vi "AdditiveChi2Sampler.vi"(8 "error in":errorcluster caption="entrée d'erreur", 11 "AdditiveChi2Sampler":T1={"sample_steps"=2, "sample_interval"=-1.0} {"sample_interval" min=-1.0}) -> (0 "error out":errorcluster caption="sortie d'erreur", 3 "AdditiveChi2Sampler.lvclass":refnum<class "AdditiveChi2Sampler.lvclass">)   [LabVIEW 2020]
doc: "Approximate feature map for additive chi2 kernel.\n\nUses sampling the fourier transform of the kernel characteristic at regular intervals.\n\nSince the kernel that is to be approximated is additive, the components of the input vectors can be treated separately. Each entry in the original space is transformed into 2*sample_steps+1 features, where sample_steps is a parameter of the method. Typical values of sample_steps include 1, 2 and 3.\n\nOptimal choices for the sampling interval for certain data ranges can be computed (see the reference). The default values should be reasonable.\n\n\nParameters : \n\n- sample_steps : int, optional=None=-1\nGives the number of (complex) sampling points.\n\n- sample_interval : float, optional=None=-1\nSampling interval. Must be specified when sample_steps not in {1,2,3}.\n\n\nMethods :\n\n- Fit : Set the parameters\n\nParameters : X : array-like, shape (n_samples, n_features)\n Training data, where n_samples in the number of samples and n_features is the number of features.\n\nReturns : String 'OK'\n\n- Fit Transform : Fit to data, then transform it.\n\nFits transformer to X and y with optional parameters fit_params and returns a transformed version of X.\n\nParameters : X : {array-like, sparse matrix, dataframe} of shape (n_samples, n_features)\n y : ndarray of shape (n_samples,), default=None\n Target values.\n\nReturns : X_new : ndarray array of shape (n_samples, n_features_new)\n Transformed array.\n\n\n- Transform : Apply approximate feature map to X.\n\nParameters : X : {array-like, sparse matrix} of shape (n_samples, n_features)\n\nReturns : X_new : {array, sparse matrix}, shape = (n_samples, n_features * (2*sample_steps + 1))\nWhether the return value is an array of sparse matrix depends on the type of the input X."
uses:
  AdditiveChi2Sampler.lvclass
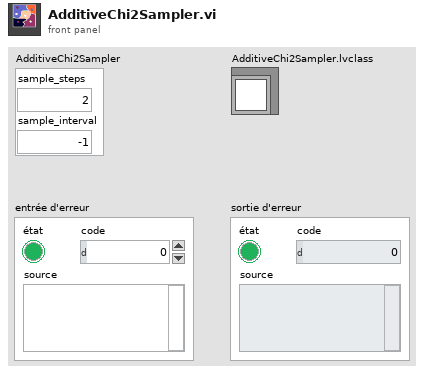
[diagram p1: front panel]
types:
  T1 = cluster{"sample_steps":i32, "sample_interval":dbl}
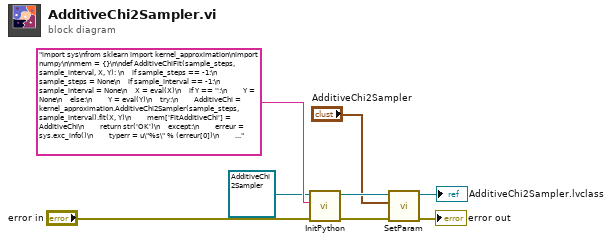
[diagram p0: block diagram]
diagram:
  n1 = call-dynamic "InitPython.vi"("error in (no error)"="error in", "Python Instruction"="import sys\nfrom sklearn import kernel_approximation\nimport numpy\n\nmem = {}\n\ndef AdditiveChiFit(sample_steps, sample_interval, X, Y): \n    if sample_steps == -1:\n        sample_steps = None\n    if sample_interval == -1:\n        sample_interval = None\n    X = eval(X)\n    if Y == '':\n        Y = None\n    else:\n        Y = eval(Y)\n    try:\n        AdditiveChi = kernel_approximation.AdditiveChi2Sampler(sample_steps, sample_interval).fit(X, Y)\n        mem['FitAdditiveChi'] = AdditiveChi\n        return str('OK')\n    except:\n        erreur = sys.exc_info()\n        typerr = u\"%s\" % (erreur[0])\n        typerr = typerr[typerr.find(\"'\")+1:typerr.rfind(\"'\")]\n        msgerr = u\"%s\" % (erreur[1])\n        message = str('/!\\\\ {0} : {1}'. format(typerr,msgerr))\n        return message \n\ndef AdditiveChiFitTransform(sample_steps, sample_interval, X, Y):\n    if sample_steps == -1:\n        sample_steps = None\n    if sample_interval == -1:\n        sample_interval = None\n    X = eval(X)\n    if Y == '':\n        Y = None\n    else:\n        Y = eval(Y)\n    try:\n        AdditiveChi = kernel_approximation.AdditiveChi2Sampler(sample_steps, sample_interval).fit_transform(X, Y)\n        dtype = type(AdditiveChi)\n        if dtype == numpy.ndarray:\n            AdditiveChi = AdditiveChi.tolist()\n            return str(AdditiveChi)\n        else:\n            Mat = AdditiveChi.tocoo()\n            return str(list(zip(Mat.row, Mat.col, Mat.data)))\n    except:\n        erreur = sys.exc_info()\n        typerr = u\"%s\" % (erreur[0])\n        typerr = typerr[typerr.find(\"'\")+1:typerr.rfind(\"'\")]\n        msgerr = u\"%s\" % (erreur[1])\n        message = str('/!\\\\ {0} : {1}'. format(typerr,msgerr))\n        return message \n    \n\ndef AdditiveChiTransform(sample_steps, sample_interval, X, Y):\n    if sample_steps == -1:\n        sample_steps = None\n    if sample_interval == -1:\n        sample_interval = None\n    X = eval(X)\n    if Y == '':\n        Y = None\n    else:\n        Y = eval(Y)\n    try:\n        AdditiveChi = mem['FitAdditiveChi'].transform(X, Y)\n        dtype = type(AdditiveChi)\n        if dtype == numpy.ndarray:\n            AdditiveChi = AdditiveChi.tolist()\n            return str(AdditiveChi)\n        else:\n            Mat = AdditiveChi.tocoo()\n            return str(list(zip(Mat.row, Mat.col, Mat.data)))\n    except:\n        erreur = sys.exc_info()\n        typerr = u\"%s\" % (erreur[0])\n        typerr = typerr[typerr.find(\"'\")+1:typerr.rfind(\"'\")]\n        msgerr = u\"%s\" % (erreur[1])\n        message = str('/!\\\\ {0} : {1}'. format(typerr,msgerr))\n        return message", "Scikit-learn en entrée"=refnum<class "AdditiveChi2Sampler.lvclass"> refnum ("AdditiveChi2Sampler.lvclass")) -> ("error out"=w4:errorcluster, "Scikit-learn en sortie"=w5:refnum<class "AdditiveChi2Sampler.lvclass">)  [unwired: 7 in]
  n2 = call-dynamic "SetParam.vi"("error in (no error)"=w4, "AdditiveChi2Sampler"="AdditiveChi2Sampler", "AdditiveChi2Sampler.lvclass"=w5) -> ("error out"=→"error out":errorcluster, "AdditiveChi2Sampler.lvclass"=→"AdditiveChi2Sampler.lvclass":refnum<class "AdditiveChi2Sampler.lvclass">)  [unwired: 7 in]
